vi "HandleTCP.vi"(8 "error in (no error)":errorcluster, 11 "connection ID":refnum<k5>) -> (0 "error out":errorcluster)   [LabVIEW 2014]
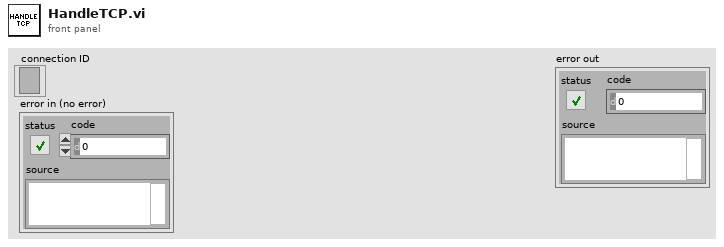
[diagram p1: front panel]
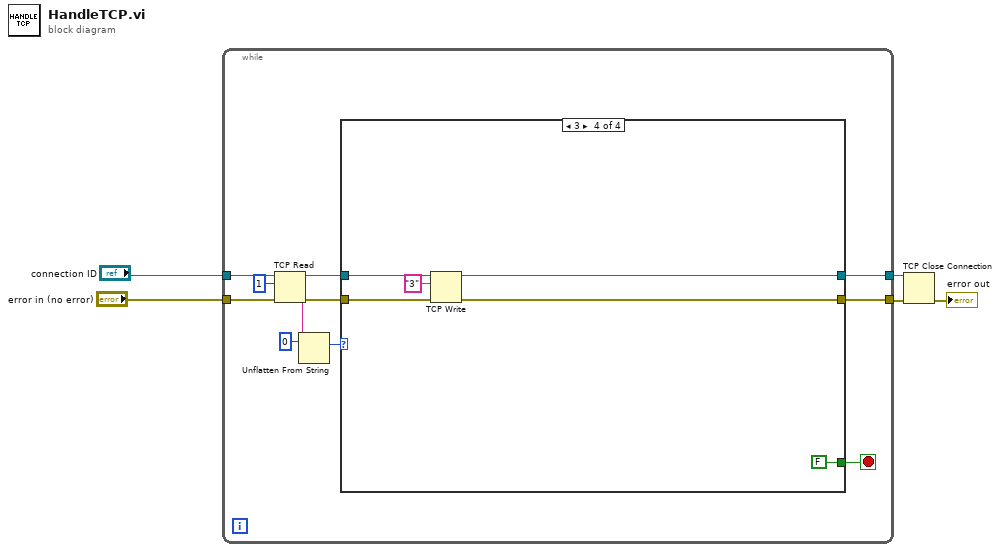
[diagram p0: block diagram]
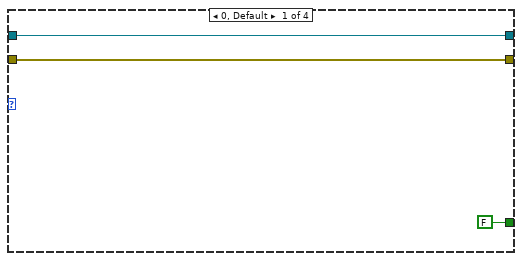
[diagram p2: hidden frame]
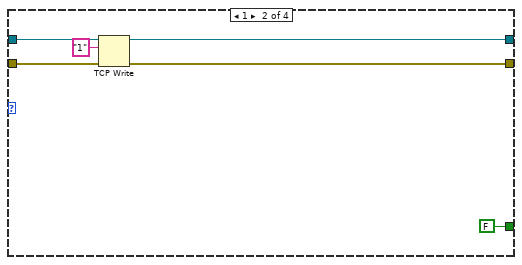
[diagram p3: hidden frame]
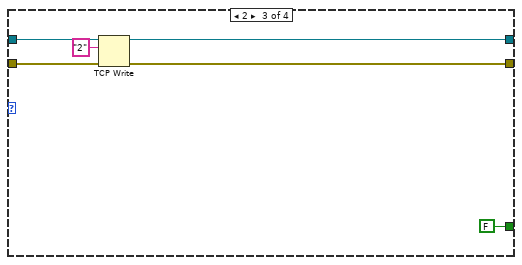
[diagram p4: hidden frame]
diagram:
  n1 = while {
    tunnel: "connection ID" -> [w15]
    tunnel: "error in (no error)" -> [w14]
    tunnel: [w7] -> w2
    tunnel: [w6] -> w3
    stop <- w8 stop-if-true
    n2 = TCP Read(connection ID=w15, bytes to read=1, error in (no error)=w14) -> (connection ID out=w12:refnum<k5>, data out=w10:string, error out=w13:errorcluster)  [unwired: 2 in]
    n3 = Unflatten From String(type=u8 0, binary string=w10) -> (value=w9:u8)  [unwired: 3 in, 2 out]
    n4 = case shown="3" w9 {
      tunnel: w13 -> [w18 w25 w31 w37]
      tunnel: w12 -> [w19 w24 w30 w36]
      tunnel: [w19 w22 w28 w34] -> w6
      tunnel: [w18 w23 w29 w35] -> w7
      tunnel: [FALSE FALSE FALSE FALSE] -> w8
      frame 0, Default {
      }
      frame 1 {
        n5 = TCP Write(connection ID=w24, data in="1", error in (no error)=w25) -> (connection ID out=w22:refnum<k5>, error out=w23:errorcluster)  [unwired: 1 in, 1 out]
      }
      frame 2 {
        n6 = TCP Write(connection ID=w30, data in="2", error in (no error)=w31) -> (connection ID out=w28:refnum<k5>, error out=w29:errorcluster)  [unwired: 1 in, 1 out]
      }
      frame 3 {
        n7 = TCP Write(connection ID=w36, data in="3", error in (no error)=w37) -> (connection ID out=w34:refnum<k5>, error out=w35:errorcluster)  [unwired: 1 in, 1 out]
      }
    }
  }
  n8 = TCP Close Connection(connection ID=w3, error in (no error)=w2) -> (error out=→"error out":errorcluster)  [unwired: 1 in, 1 out]
